vi "ConvertMatlabDataValueToVartiant.vi"(9 "Allow Variant Values (f)":bool, 10 "MatlabDataBundle":T1, 11 "Data Value":variant) -> (3 "Value":variant)   [LabVIEW 2017]
uses:
  Types/MatlabDataBundle.ctl
  Types/MatlabDataType.ctl
  Types/MatlabDataContainerType.ctl
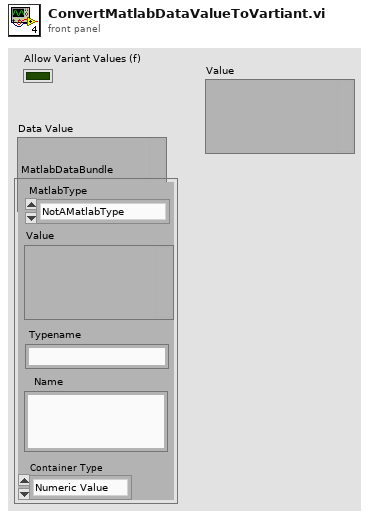
[diagram p1: front panel]
types:
  T1 = typedef "MatlabDataBundle.ctl" = cluster{"MatlabType":T2, "Value":variant, "Name":string, "Typename":string, "Container Type":T3}
  T2 = typedef "MatlabDataType.ctl" = enum16{"NotAMatlabType", "Real", "Complex", "String", "Boolean"}
  T3 = typedef "MatlabDataContainerType.ctl" = enum16{"Numeric Value", "Numeric Array", "Waveform"}
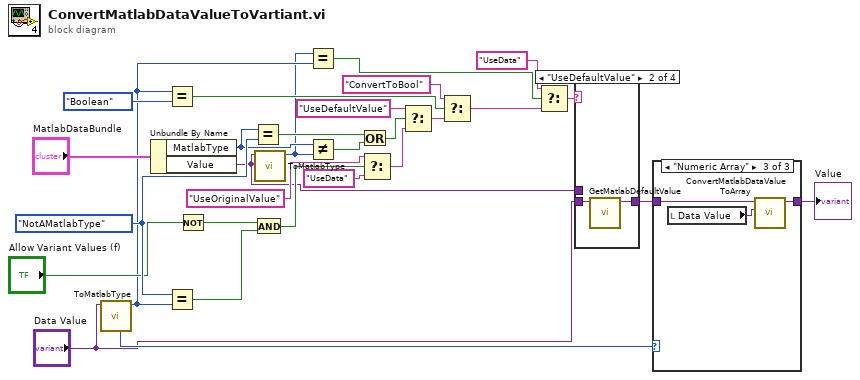
[diagram p0: block diagram]
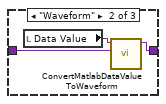
[diagram p3: hidden frame]
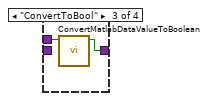
[diagram p5: hidden frame]
diagram:
  w20 = MatlabDataType."NotAMatlabType" ("MatlabType")
  n1 = call "ToMatlabType.vi"("Value"="Data Value") -> ("MatlabType"=w10:T2, "Container Type (Labview Value type)"=w9:T3)  [unwired: 6 in, 3 out]
  n2 = Unbundle By Name("MatlabDataBundle") -> ("MatlabType"=w7:T2, "Value"=w4:variant)
  n3 = Equal?(x=w10, y=MatlabDataType."Boolean" ("MatlabType")) -> (x = y?=w25:bool)
  n4 = Equal?(x=w20, y=w10) -> (x = y?=w17:bool)
  n5 = Not(x="Allow Variant Values (f)") -> (.not. x?=w19:bool)
  n6 = Equal?(x=w7, y=w20) -> (x = y?=w21:bool)
  n7 = And(x=w19, y=w17) -> (x .and. y?=w16:bool)
  n8 = call "ToMatlabType.vi"("Value"=w4) -> ("MatlabType"=w1:T2)  [unwired: 6 in, 4 out]
  n9 = Equal?(x=w1, y=w10) -> (x = y?=w27:bool)
  n10 = Not Equal?(x=w7, y=w1) -> (x != y?=w5:bool)
  n11 = Or(x=w21, y=w5) -> (x .or. y?=w6:bool)
  n12 = Select(t="UseOriginalValue", s=w16, f="UseData") -> (s? t:f=w14:string)
  n13 = Select(t="UseDefaultValue", s=w6, f=w14) -> (s? t:f=w22:string)
  n14 = Select(t="ConvertToBool", s=w25, f=w22) -> (s? t:f=w24:string)
  n15 = Select(t="UseData", s=w27, f=w24) -> (s? t:f=w29:string)
  n16 = case shown="\"UseDefaultValue\"" w29 {
    tunnel: w4 -> [w30 _ w33 _]
    tunnel: [w30 w32 w34 w35] -> w12
    tunnel: "Data Value" -> [_ w31 _ w35]
    frame Default {
    }
    frame "UseDefaultValue" {
      n17 = call "GetMatlabDefaultValue.vi"("From Value Type"=w31) -> ("Default Value"=w32:variant)  [unwired: 10 in]
    }
    frame "ConvertToBool" {
      n18 = call "ConvertMatlabDataValueToBoolean.vi"("Data Value"=w33) -> ("Boolean"=w34:bool)  [unwired: 10 in]
    }
    frame "UseOriginalValue" {
    }
  }
  n19 = case shown="\"Numeric Array\"" w9 {
    tunnel: w12 -> [w36 w39 w41]
    tunnel: [w36 w37 w42] -> w11
    frame Default {
    }
    frame "Waveform" {
      n20 = local read "Data Value"() -> (w38:variant)
      n21 = call "ConvertMatlabDataValueToWaveform.vi"("Numbers Vector"=w39, "Waveform"=w38) -> ("Data Value out"=w37:variant)  [unwired: 9 in]
    }
    frame "Numeric Array" {
      n22 = local read "Data Value"() -> (w40:variant)
      n23 = call "ConvertMatlabDataValueToArray.vi"("Original Value"=w40, "Data"=w41) -> ("Array"=w42:variant)  [unwired: 9 in]
    }
  }
  "Value" <- w11
